vi "main.vi"() -> ()   [LabVIEW 2020]
panel:
  in  "NumElements":dbl=5.0
  in  "End":dbl=20.0
  in  "Start":dbl
  in  "Number of iterations":dbl
  out "Mandelbrot set by Adam Ignaciuk":i32[][](graph)
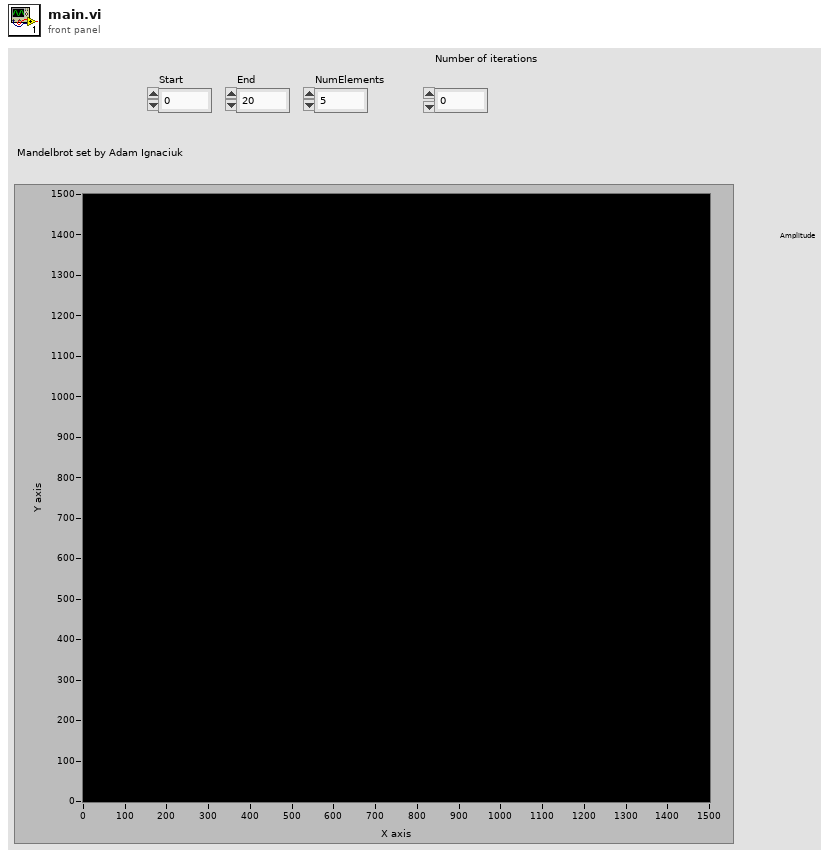
[diagram p1: front panel]
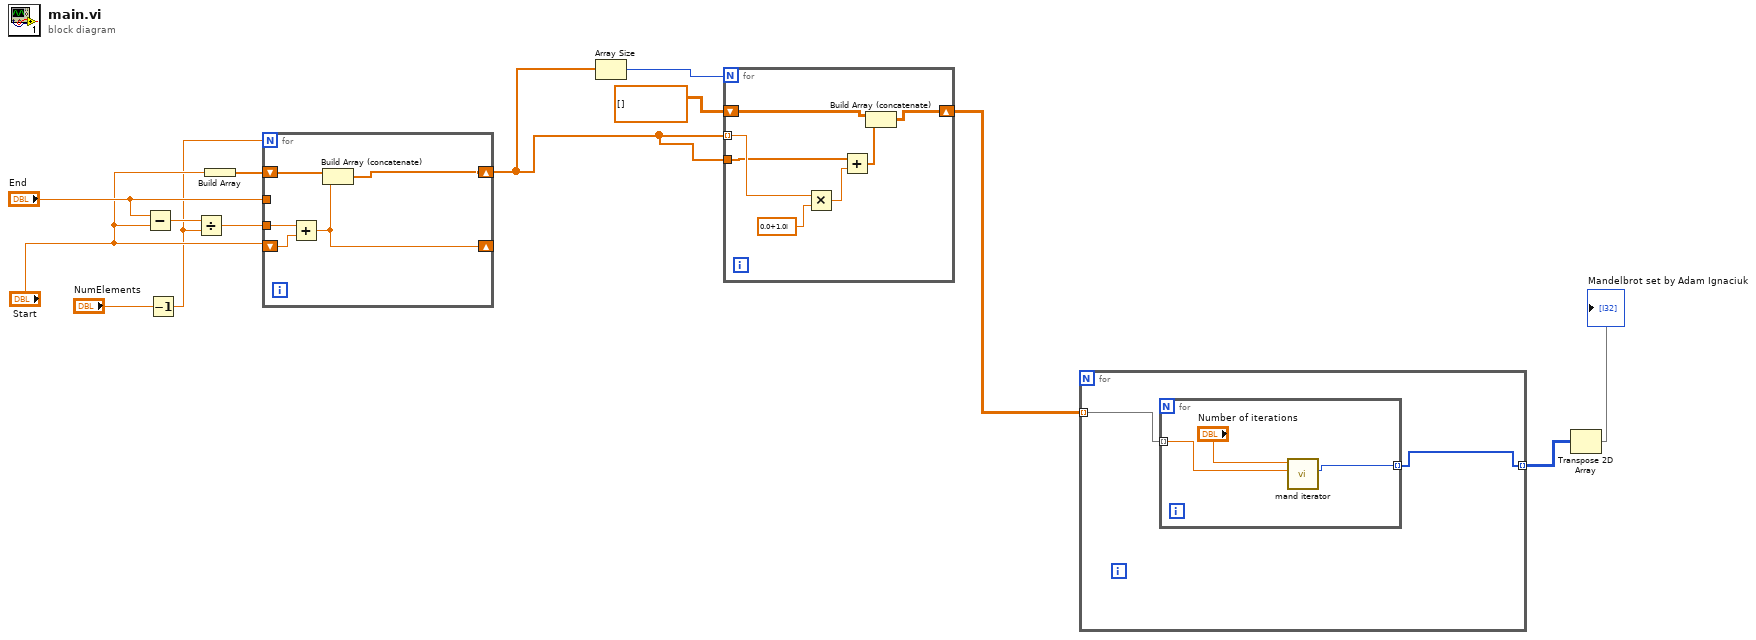
[diagram p0: block diagram]
diagram:
  n1 = Subtract(x="End", y="Start") -> (x-y=w13:dbl)
  n2 = Decrement(x="NumElements") -> (x-1=w7:dbl)
  n3 = Divide(x=w13, y=w7) -> (x/y=w12:dbl)
  n4 = Build Array("Start") -> (w10:dbl[])
  n5 = for {
    N: w7 -> [_]
    shift-right: [w15] -> w5
    shift-left: w10 -> [w18]
    tunnel: w12 -> [w17]
    tunnel: "End" -> [_]
    shift-right: [w14] -> _
    shift-left: "Start" -> [w16]
    n6 = Add(x=w17, y=w16) -> (x+y=w14:dbl)
    n7 = Build Array (concatenate)(w18, w14) -> (w15:dbl[])
  }
  n8 = Array Size(array=w5) -> (size(s)=w6:i32)
  n9 = for {
    N: w6 -> [_]
    tunnel: w5 -> [w24] mode=indexing
    tunnel: w5 -> [w23]
    shift-right: [w19] -> w3
    shift-left: cdb[][] [] -> [w21]
    n10 = Multiply(x=w24, y=csg 0.0+1.0i) -> (x*y=w22:cdb)
    n11 = Add(x=w23, y=w22) -> (x+y=w20:cdb[])
    n12 = Build Array (concatenate)(w21, w20) -> (w19:cdb[][])
  }
  n13 = for {
    tunnel: w3 -> [w27] mode=indexing
    tunnel: [w26] -> w2 mode=indexing
    n14 = for {
      tunnel: w27 -> [w29] mode=indexing
      tunnel: [w28] -> w26 mode=indexing
      n15 = call "mand iterator.vi"("C"=w29, "Number of iterations"="Number of iterations") -> ("Z out"=w28:i32)  [unwired: 9 in]
    }
  }
  n16 = Transpose 2D Array(2D array=w2) -> (transposed array=→"Mandelbrot set by Adam Ignaciuk":i32[][])
